vi "DSP.TestLauncher.vi"() -> ()   [LabVIEW 2016, in "DSP.lvclass"]
uses:
  DSP.lvclass
  <vilib>/JKI/JKI SMO/SMO/Typedefs/SMOState --Enum.ctl
  Typedefs/LP_Config.ctl
  DSP.lockin/Typedefs/Lockin_Config.ctl
  Typedefs/FFT_Config.ctl
  <vilib>/Analysis/4window.llb/windowTd.ctl
  <vilib>/measure/maspectr.llb/Power Spectrum and PSD Export Mode.ctl
  lockin/Typedefs/output_config.ctl
  C:/Program Files (x86)/National Instruments/LabVIEW 2016/vi.lib/JKI/JKI SMO/SMO/SMO.lvclass
  <vilib>/JKI/JKI SMO/SMO/SMO.lvclass
  lockin/lockin.lvclass
  DSP.lockin/DSP_lockin.lvclass
  <vilib>/Analysis/NI_AALPro.lvlib
  <vilib>/measure/NI_MAPro.lvlib
panel:
  in  "display Waveforms":bool
  in  "sampling info":cluster{"Fs":dbl, "#s":dbl}={"Fs"=1000.0, "#s"=1000.0} {"Fs" format="%.2p"}
  out "getLockin":dbl[][](graph)
  in  "do calculation":bool
  in  "output config":T1=[{"A (V)"=1.0, "DC (V)"=0.0, "f (Hz)"=1.0, "phi (deg)"=0.0, "signal type"=enum."Sine Wave"}, {"A (V)"=2.0, "DC (V)"=0.0, "f (Hz)"=2.0, "phi (deg)"=0.0, "signal type"=enum."Sine Wave"}, {"A (V)"=3.0, "DC (V)"=0.0, "f (Hz)"=3.0, "phi (deg)"=0.0, "signal type"=enum."Sine Wave"}, {"A (V)"=4.0, "DC (V)"=0.0, "f (Hz)"=4.0, "phi (deg)"=0.0, "signal type"=enum."Sine Wave"}, {"A (V)"=5.0, "DC (V)"=0.0, "f (Hz)"=5.0, "phi (deg)"=0.0, "signal type"=enum."Sine Wave"}, {"A (V)"=6.0, "DC (V)"=0.0, "f (Hz)"=6.0, "phi (deg)"=0.0, "signal type"=enum."Sine Wave"}, {"A (V)"=7.0, "DC (V)"=0.0, "f (Hz)"=7.0, "phi (deg)"=0.0, "signal type"=enum."Sine Wave"}]
  in  "update waveform":bool
  out "getWaveforms":T2(graph)
  out "getPowerSpectrum":T3(graph)
  in  "RunCalculation":T9 {"RunCalculation"."FFT config"."export mode" items=["Power Spectrum", "Power Spectral Density"]; "RunCalculation"."FFT config"."window" items=["Rectangle"=0, "Hanning"=1, "Hamming"=2, "Blackman-Harris"=3, "Exact Blackman"=4, "Blackman"=5, "Flat Top"=6, "4 Term B-Harris "=7, "7 Term B-Harris"=8, "Low Sidelobe"=9, "Blackman Nuttall"=11, "Triangle"=30, "Bartlett-Hanning"=31, "Bohman"=32, "Parzen"=33, "Welch"=34, "Kaiser"=60, "Dolph-Chebyshev"=61, "Gaussian"=62]; "RunCalculation"."FFT config"."averaging parameters"."number of averages" min=1; "RunCalculation"."Lockin config"."TC (s)" format="%#_13g"}
  out "SMO State":T10
  out "error out":errorcluster
  in  "Stop":bool
  # "Basic SMO Test Launcher"
  # "For instructions on how to use the JKI State Machine Objects, examples and video tutorials, visit:\nhttp://jki.net/state-machine-objects/\n\nJKI State Machine Objects™\nhttp://jki.net/state-machine-objects/\nCopyright (C) 2005-2015, JKI <info@jki.net>\nALL RIGHTS RESERVED"
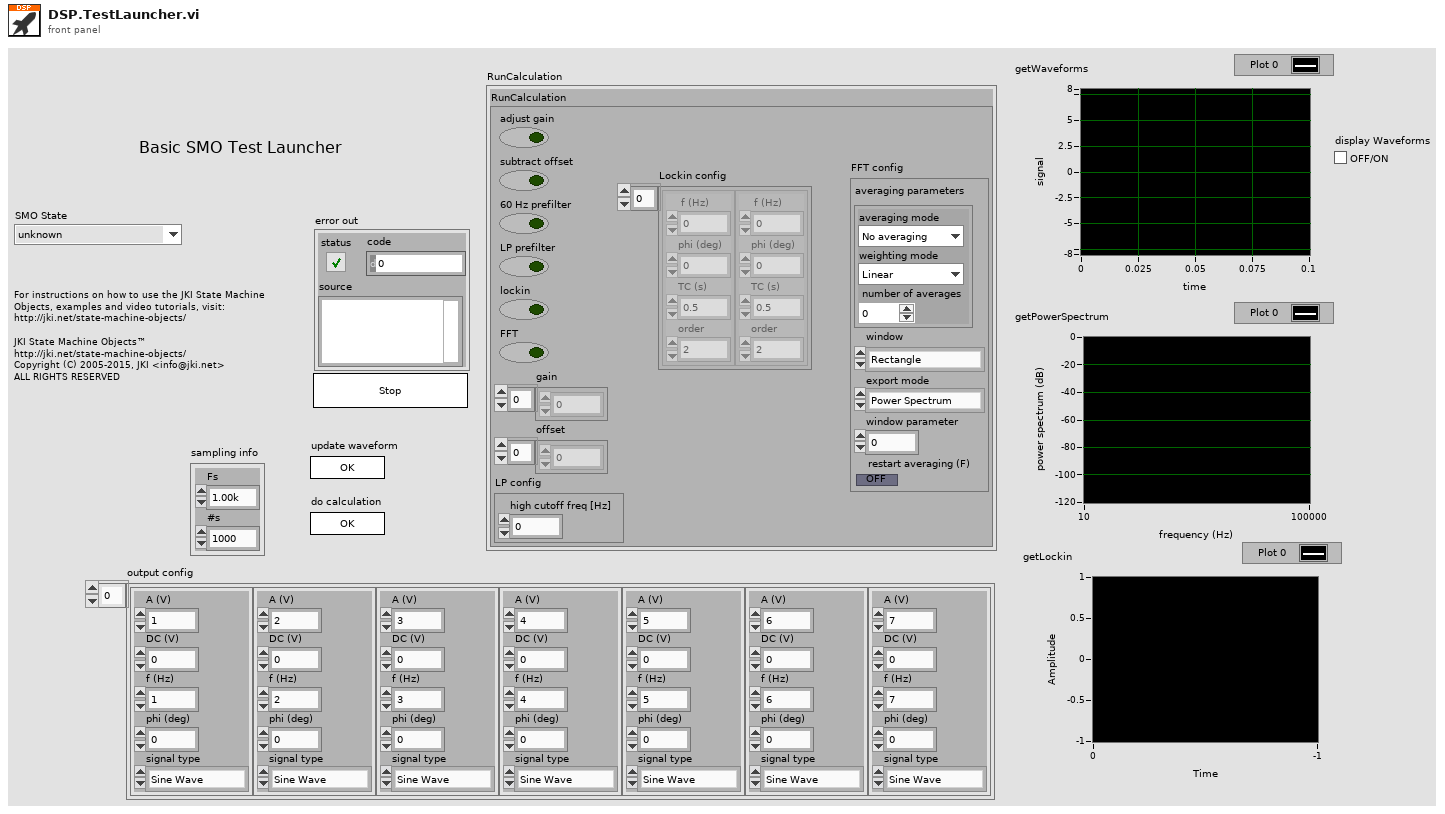
[diagram p1: front panel]
types:
  T1 = typedef "lockin.lvclass/output_config.ctl" = cluster{"A (V)":dbl, "DC (V)":dbl, "f (Hz)":dbl, "phi (deg)":dbl, "signal type":enum16{"Sine Wave", "Triangle Wave", "Square Wave", "Sawtooth Wave"}}[]
  T2 = typedef "PublicEvents--DSP.getWaveforms.ctl" = waveform(dbl)[]
  T3 = typedef "DSP.lvclass/PublicEvents--DSP.getPowerSpectrum.ctl" = cluster{"f0":dbl, "df":dbl, "magnitude":dbl[]}[]
  T4 = typedef "DSP.lvclass/LP_Config.ctl" = cluster{"high cutoff freq [Hz]":dbl}
  T5 = typedef "DSP_lockin.lvclass/Lockin_Config.ctl" = cluster{" f (Hz)":dbl, "phi (deg)":dbl, "TC (s)":dbl, "order":i32}[]
  T6 = typedef "DSP.lvclass/FFT_Config.ctl" = cluster{"averaging parameters":cluster{"averaging mode":enum16{"No averaging", "Vector averaging", "RMS averaging", "Peak hold"}, "weighting mode":enum16{"Linear", "Exponential"}, "number of averages":u32}, "window":T7, "export mode":T8, "window parameter":dbl, "restart averaging (F)":bool}
  T7 = typedef "NI_AALPro.lvlib/windowTd.ctl" = u32
  T8 = typedef "NI_MAPro.lvlib/Power Spectrum and PSD Export Mode.ctl" = u16
  T9 = cluster{"RunCalculation":cluster{"adjust gain":bool, "subtract offset":bool, "60 Hz prefilter":bool, "LP prefilter":bool, "lockin":bool, "FFT":bool, "gain":dbl[], "offset":dbl[], "LP config":T4, "Lockin config":T5, "FFT config":T6}}
  T10 = typedef "SMO.lvclass/SMOState --Enum.ctl" = enum16{"unknown", "Created", "Started", "Stopped"}
  T11 = typedef "SMO.lvclass/Public Events.ctl" = cluster{"Error":refnum<user-event>, "State":refnum<user-event>, "Reserve State":refnum<user-event>}
  T12 = typedef "DSP.lvclass/PublicEvents--Cluster.ctl" = cluster{"getWaveforms":refnum<user-event>, "getLockin":refnum<user-event>, "getPowerSpectrum":refnum<user-event>}
  T13 = cluster{"Event Registration Refnum":refnum<event-registration>}
  T14 = typedef "DSP.lvclass/PublicEvents--DSP.getLockin.ctl" = T15[]
  T15 = typedef "DSP_lockin.lvclass/LockinResult.ctl" = cluster{"X":dbl, "Y":dbl, "R":dbl, "Theta":dbl, "AVG":dbl, "f":dbl, "Name":string}
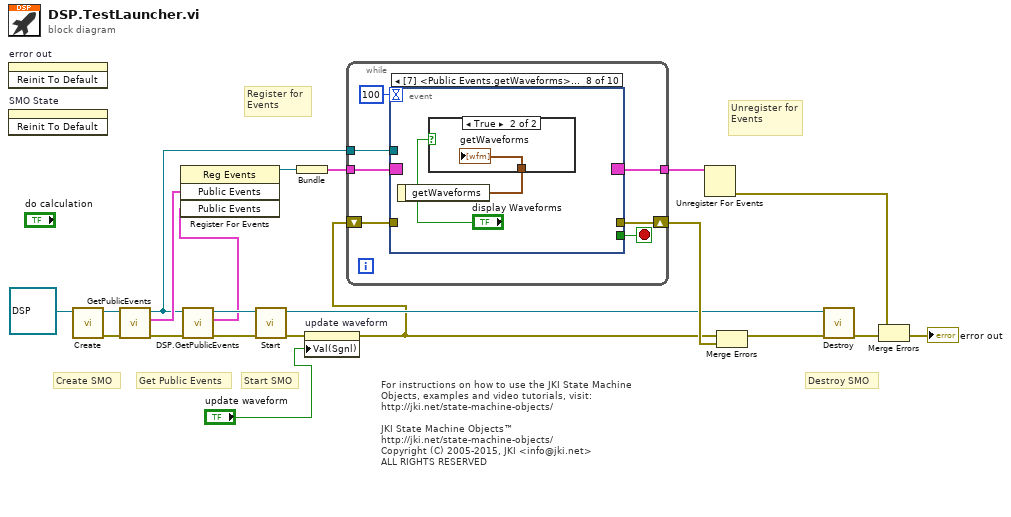
[diagram p0: block diagram]
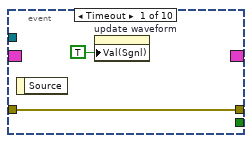
[diagram p2: hidden frame]
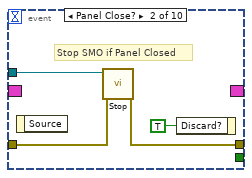
[diagram p3: hidden frame]
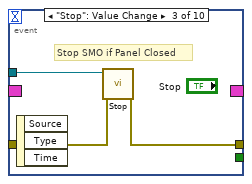
[diagram p4: hidden frame]
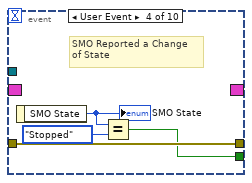
[diagram p5: hidden frame]
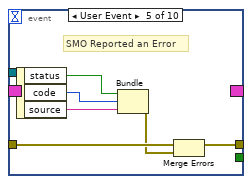
[diagram p6: hidden frame]
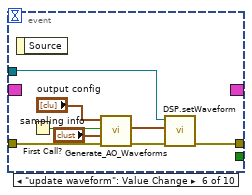
[diagram p7: hidden frame]
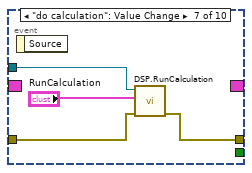
[diagram p8: hidden frame]
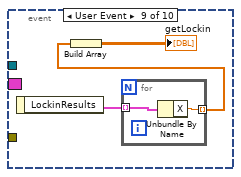
[diagram p10: hidden frame]
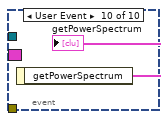
[diagram p11: hidden frame]
diagram:
  # "For instructions on how to use the JKI State Machine Objects, examples and video tutorials, visit:\nhttp://jki.net/state-machine-objects/\n\nJKI State Machine Objects™\nhttp://jki.net/state-machine-objects/\nCopyright (C) 2005-2015, JKI <info@jki.net>\nALL RIGHTS RESERVED"
  # "Get Public Events"
  # "Start SMO"
  # "Destroy SMO"
  # "Create SMO"
  # "Unregister for Events"
  # "Register for Events"
  n1 = invoke on="error out" class="Clust (strict)" method="Reinit To Default"() -> ()  [unwired: 3 in, 3 out]
  n2 = invoke on="SMO State" class="Enum (strict)" method="Reinit To Default"() -> ()  [unwired: 3 in, 3 out]
  n3 = call <vilib>:"Create.vi"("SMO"=refnum<class "DSP.lvclass"> refnum ("SMO.Template.lvclass")) -> ("error out"=w11:errorcluster, "SMO out"=w12:refnum<class "DSP.lvclass">)  [unwired: 8 in, 1 out]
  n4 = call <vilib>:"GetPublicEvents.vi"("error in (no error)"=w11, "SMO"=w12) -> ("error out"=w8:errorcluster, "Public Events"=w10:T11, "SMO out"=w7:refnum<class "DSP.lvclass">)  [unwired: 7 in]
  n5 = call "DSP.GetPublicEvents.vi"("error in (no error)"=w8, "DSP"=w7) -> ("error out"=w5:errorcluster, "Public Events"=w4:T12, "DSP out"=w6:refnum<class "DSP.lvclass">)  [unwired: 7 in]
  n6 = register-events(w10, w4) -> (reference out=w9:refnum<event-registration>)  [unwired: 2 in, 1 out]
  n7 = call <vilib>:"Start.vi"("error in (no error)"=w5, "SMO"=w6) -> ("error out"=w3:errorcluster, "SMO out"=w13:refnum<class "DSP.lvclass">)  [unwired: 8 in]
  n8 = Bundle("Event Registration Refnum"=w9) -> (w20:T13)  [unwired: 1 in]
  n9 = property on="update waveform" class="Bool (strict)"(error in=w3, "Val(Sgnl)"="update waveform") -> (error out=w2:errorcluster)  [unwired: 1 in, 1 out]
  n10 = while {
    shift-right: [w27] -> w19
    shift-left: w2 -> [w26]
    tunnel: w20 -> [w25]
    tunnel: [w24] -> w21
    tunnel: w7 -> [w23]
    stop <- w28 stop-if-true
    n11 = event shown="[7] <Public Events.getWaveforms>: User Event" {
      selector: w25 -> [_ _ _ _ _ _ _ _ _ _]
      dyn-events: [_ _ _ _ _ _ _ _ _ _] -> w24
      timeout: 100 -> [_ _ _ _ _ _ _ _ _ _]
      tunnel: [_ _ _ w38 _ _ _ _ _ _] -> w28
      tunnel: w23 -> [_ w34 w37 _ _ w54 w59 _ _ _]
      tunnel: [w30 w33 w36 w41 w45 w55 w56 _ _ _] -> w27
      tunnel: w26 -> [w30 w32 w35 w41 w43 w53 w57 _ _ _]
      event Timeout {
        n12 = event-data() -> ()  [unwired: 1 in, 1 out]
        n13 = property on="update waveform" class="Bool (strict)"("Val(Sgnl)"=TRUE ("Value (Signaling)")) -> ()  [unwired: 2 in, 2 out]
      }
      event Panel Close? {
        # "Stop SMO if Panel Closed"
        n14 = event-data() -> ()  [unwired: 1 in, 1 out]
        n15 = call <vilib>:"Stop.vi"("error in (no error)"=w32, "SMO"=w34) -> ("error out"=w33:errorcluster)  [unwired: 8 in, 1 out]
        n16 = event-data("Discard?"=TRUE ("OK")) -> ()  [unwired: 1 in, 1 out]
      }
      event "Stop": Value Change {
        # "Stop SMO if Panel Closed"
        n17 = event-data() -> ()  [unwired: 1 in, 3 out]
        n18 = call <vilib>:"Stop.vi"("error in (no error)"=w35, "SMO"=w37) -> ("error out"=w36:errorcluster)  [unwired: 8 in, 1 out]
      }
      event User Event {
        # "SMO Reported a Change\nof State"
        n19 = event-data() -> ("SMO State"=w40:T10)  [unwired: 1 in]
        "SMO State" <- w40
        n20 = Equal?(x=w40, y=SMOState_--Enum."Stopped") -> (x = y?=w38:bool)
      }
      event User Event {
        # "SMO Reported an Error"
        n21 = event-data() -> ("status"=w44:bool, "code"=w47:i32, "source"=w46:string)  [unwired: 1 in]
        n22 = Bundle("status"=w44, "code"=w47, "source"=w46) -> (w42:errorcluster)  [unwired: 1 in]
        n23 = Merge Errors(w43, w42) -> (w45:errorcluster)
      }
      event "update waveform": Value Change {
        n24 = event-data() -> ()  [unwired: 1 in, 1 out]
        n25 = First Call?() -> (First Call?: T/F=w50:bool)
        n26 = call "Generate_AO_Waveforms.vi"("error in (no error)"=w53, "sampling info"="sampling info", "reset signal"=w50, "output config"="output config") -> ("error out"=w52:errorcluster, "AO Array"=w51:waveform(dbl)[])  [unwired: 6 in]
        n27 = call "DSP.setWaveform.vi"("error in (no error)"=w52, "setWaveform"=w51, "DSP"=w54) -> ("error out"=w55:errorcluster)  [unwired: 7 in, 1 out]
      }
      event "do calculation": Value Change {
        n28 = event-data() -> ()  [unwired: 1 in, 1 out]
        n29 = call "DSP.RunCalculation.vi"("error in (no error)"=w57, "RunCalculation"="RunCalculation", "DSP"=w59) -> ("error out"=w56:errorcluster)  [unwired: 7 in, 1 out]
      }
      event User Event {
        n30 = event-data() -> ("getWaveforms"=w61:T2)  [unwired: 1 in]
        n31 = case shown="True" "display Waveforms" {
          tunnel: w61 -> [_ w62]
          frame False {
          }
          frame True {
            "getWaveforms" <- w62
          }
        }
      }
      event User Event {
        n32 = event-data() -> ("LockinResults"=w64:T14)  [unwired: 1 in]
        n33 = for {
          tunnel: [w67] -> w65 mode=indexing
          tunnel: w64 -> [w66] mode=indexing
          n34 = Unbundle By Name(w66) -> ("X"=w67:dbl)
        }
        n35 = Build Array(w65) -> (→"getLockin":dbl[][])
      }
      event User Event {
        n36 = event-data() -> ("getPowerSpectrum"=→"getPowerSpectrum":T3)  [unwired: 1 in]
      }
    }
  }
  n37 = Unregister For Events(event registration refnum=w21) -> (error out=w18:errorcluster)  [unwired: 1 in]
  n38 = Merge Errors(w2, w19) -> (w14:errorcluster)
  n39 = call <vilib>:"Destroy.vi"("error in (no error)"=w14, "SMO"=w13) -> ("error out"=w16:errorcluster)  [unwired: 9 in]
  n40 = Merge Errors(w18, w16) -> (→"error out":errorcluster)
